vi "Basic Graph.vi"() -> ()   [LabVIEW 2014]
uses:
  <vilib>/measure/NI_MABase.lvlib
panel:
  in  "Frequency":dbl(knob) scale=0.0..10.0
  in  "Amplitude":dbl(knob) scale=0.0..10.0
  in  "stop":bool
  out "Waveform Graph":waveform(dbl)(graph)
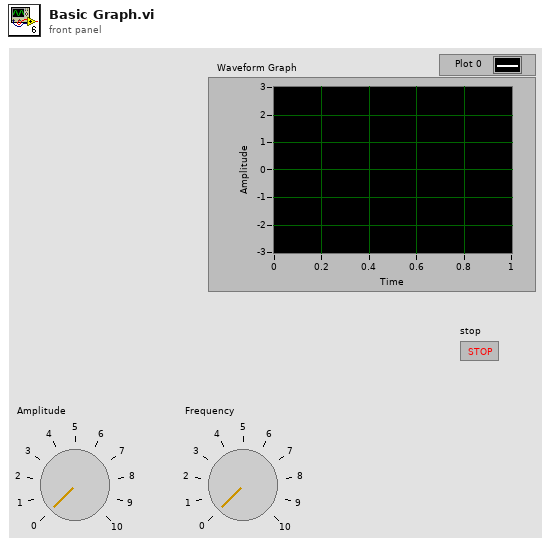
[diagram p1: front panel]
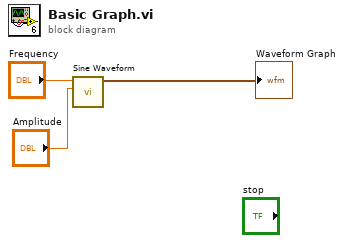
[diagram p0: block diagram]
diagram:
  n1 = call <vilib>:"Sine Waveform.vi"("amplitude"="Amplitude", "frequency"="Frequency") -> ("signal out"=→"Waveform Graph":waveform(dbl))  [unwired: 8 in, 1 out]
